vi "Run Vi.vi"(0 "Bring To Front (T)":bool=TRUE, 2 "VI Path":path, 3 "error in (no error)":errorcluster, 4 "Start Hidden? (F)":bool, 8 "Activate? (T)":bool=TRUE) -> (7 "Window State":T1(ring), 9 "error out":errorcluster)   [LabVIEW 2021, in "Utilities.lvlib"]
uses:
  Utilities.lvlib
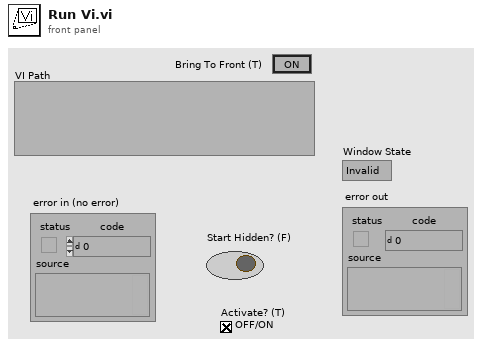
[diagram p1: front panel]
types:
  T1 = enum32{"Invalid", "Standard", "Closed", "Hidden", "Minimized", "Maximized"}
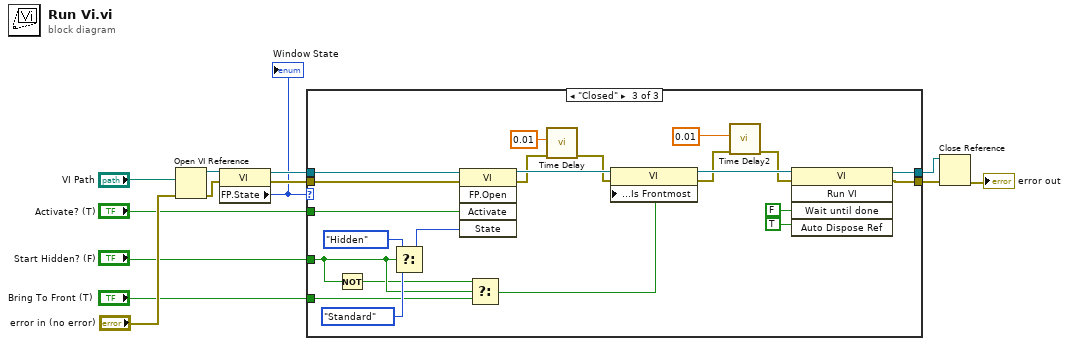
[diagram p0: block diagram]
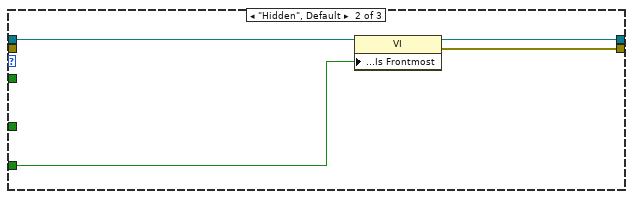
[diagram p3: hidden frame]
diagram:
  n1 = Open VI Reference(vi path="VI Path", error in (no error)="error in (no error)") -> (vi reference=w13:refnum<vi>, error out=w12:errorcluster)  [unwired: 4 in]
  n2 = property class="VI"(reference=w13, error in=w12) -> (reference out=w11:refnum<vi>, error out=w10:errorcluster, "FP.State"=w6:T1)
  "Window State" <- w6
  n3 = case shown="\"Closed\"" w6 {
    tunnel: w11 -> [w14 w19 w41]
    tunnel: w10 -> [w15 _ w33]
    tunnel: [w15 w18 w37] -> w4
    tunnel: "Bring To Front (T)" -> [_ w17 w28]
    tunnel: "Start Hidden? (F)" -> [_ _ w29]
    tunnel: [w14 w16 w25] -> w2
    tunnel: "Activate? (T)" -> [_ _ w20]
    frame "Invalid" {
    }
    frame "Hidden", Default {
      n4 = property class="VI"(reference=w19, "Front Panel Window:Is Frontmost"=w17) -> (reference out=w16:refnum<vi>, error out=w18:errorcluster)  [unwired: 1 in]
    }
    frame "Closed" {
      n5 = Not(x=w29) -> (.not. x?=w27:bool)
      n6 = Select(t=T1."Hidden" ("State"), s=w29, f=T1."Standard" ("State")) -> (s? t:f=w30:T1)
      n7 = invoke class="VI" method="FP.Open"(reference=w41, error in=w33, "Activate"=w20, "State"=w30) -> (reference out=w35:refnum<vi>, error out=w34:errorcluster)  [unwired: 1 in, 3 out]
      n8 = Select(t=w27, s=w29, f=w28) -> (s? t:f=w26:bool)
      n9 = call "Time Delay"("error in (no error)"=w34, "Delay Time (s)"=0.01) -> ("error out"=w24:errorcluster)  [unwired: 9 in]
      n10 = property class="VI"(reference=w35, error in=w24, "Front Panel Window:Is Frontmost"=w26) -> (reference out=w40:refnum<vi>, error out=w39:errorcluster)
      n11 = call "Time Delay2"("error in (no error)"=w39, "Delay Time (s)"=0.01) -> ("error out"=w22:errorcluster)  [unwired: 9 in]
      n12 = invoke class="VI" method="Run VI"(reference=w40, error in=w22, "Wait until done"=FALSE, "Auto Dispose Ref"=TRUE) -> (reference out=w25:refnum<vi>, error out=w37:errorcluster)  [unwired: 1 in, 3 out]
    }
  }
  n13 = Close Reference(reference=w2, error in (no error)=w4) -> (error out=→"error out":errorcluster)
